vi "Build KEYBDINPUT Struct.vi"(8 "error in (no error)":errorcluster, 10 "Flags":u32, 11 "Vk":u16) -> (0 "error out":errorcluster, 3 "Array":u8[](array[numeric]))   [LabVIEW 2020, in "MacroAssert.lvlib" / "Win Util.lvlib"]
uses:
  Win Util.lvlib
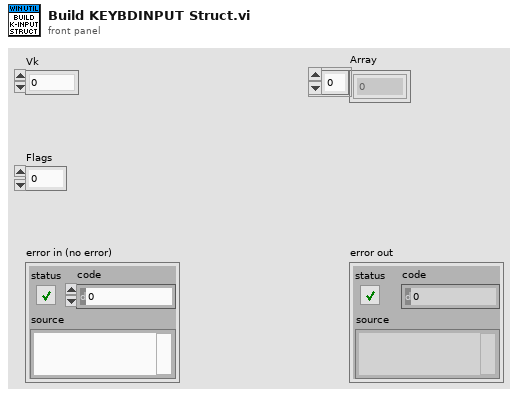
[diagram p1: front panel]
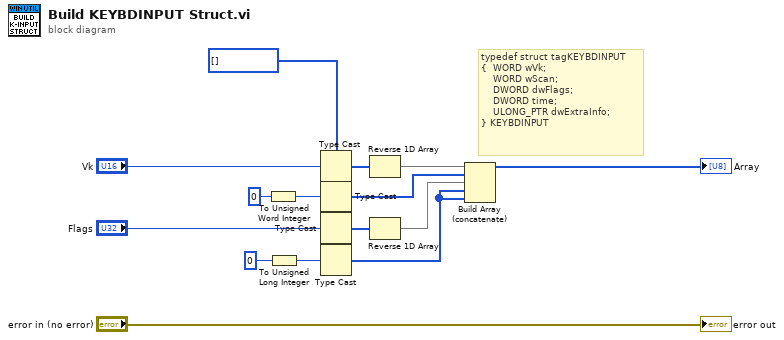
[diagram p0: block diagram]
diagram:
  w4 = u8[] []
  # "typedef struct tagKEYBDINPUT\n{  WORD wVk;\n    WORD wScan;\n    DWORD dwFlags;\n    DWORD time;\n    ULONG_PTR dwExtraInfo;\n} KEYBDINPUT"
  n1 = To Unsigned Word Integer(number=u16 0 ("Vk")) -> (unsigned 16bit integer=w12:u16)
  n2 = To Unsigned Long Integer(number=u32 0 ("Vk")) -> (unsigned 32bit integer=w5:u32)
  n3 = Type Cast(type=w4, x="Vk") -> (*(type *) &x=w10:u8[])
  n4 = Type Cast(type=w4, x=w12) -> (*(type *) &x=w8:u8[])
  n5 = Type Cast(type=w4, x="Flags") -> (*(type *) &x=w7:u8[])
  n6 = Type Cast(type=w4, x=w5) -> (*(type *) &x=w3:u8[])
  n7 = Reverse 1D Array(array=w10) -> (reversed array=w9:u8[])
  n8 = Reverse 1D Array(array=w7) -> (reversed array=w6:u8[])
  n9 = Build Array (concatenate)(w9, w8, w6, w3, w3) -> (→"Array":u8[])
  "error out" <- "error in (no error)"
